vi "test_variance_map.vi"() -> ()   [LabVIEW 2009]
doc: "Copyright (C) 2009, Stepan A. Baranov\nweb: http://www.OCTLab.org/\nemail: stepan@baranov.su"
uses:
  <vilib>/Analysis/NI_AALBase.lvlib
  OCTLib.dll
panel:
  out "vertical radius":i32
  out "error out":errorcluster
  out "horizontal radius":i32
  out "width":i32
  out "height":i32
  in  "Small/Big":bool
  out "loop #":i32
  out "RSM_STAT time":u32
  out "LabView time":u32
  out "RSM_STAT Array":dbl[][](array[numeric])
  out "LabView Array":dbl[][](array[numeric])
  in  "stop":bool
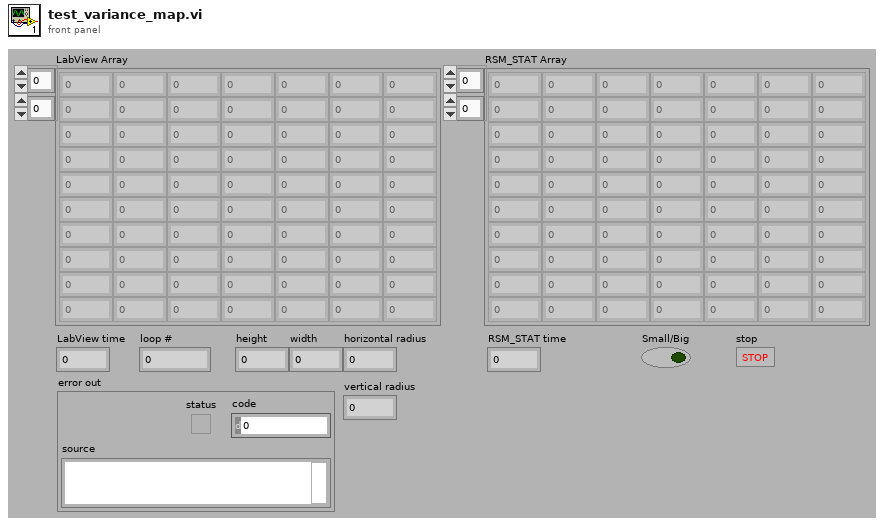
[diagram p1: front panel]
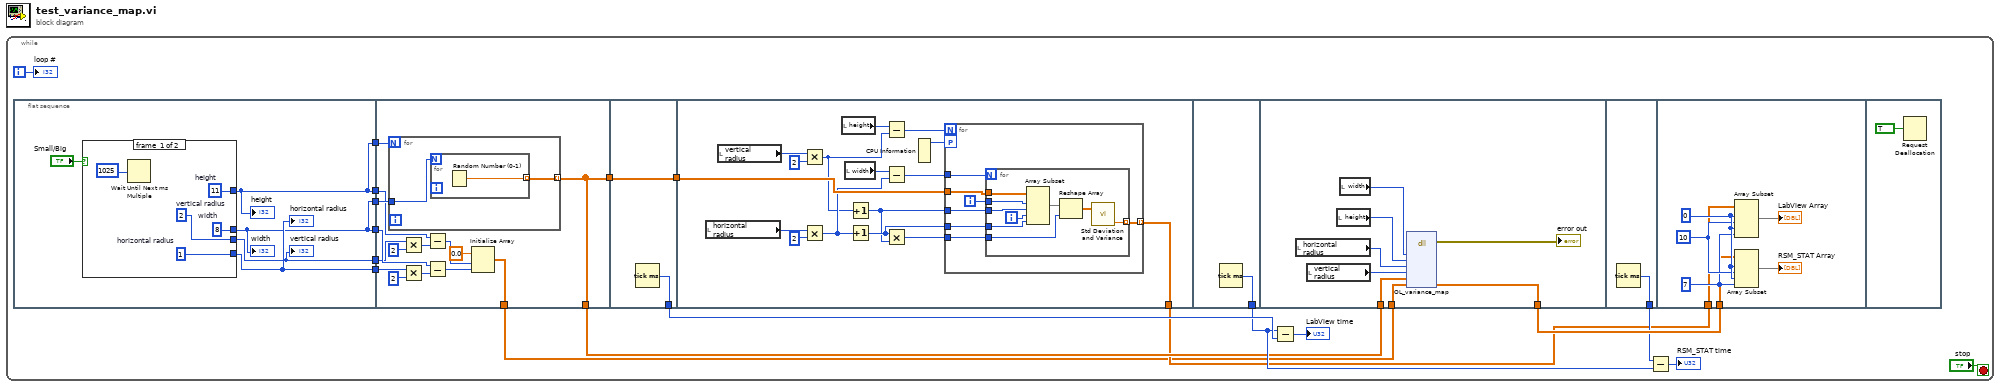
[diagram p0: block diagram]
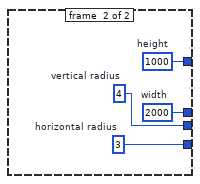
[diagram p2: hidden frame]
diagram:
  n1 = while {
    i -> [w12]
    stop <- "stop" stop-if-true
    n2 = flat-sequence {
      tunnel: [w21] -> w8
      tunnel: [w22] -> w7
      tunnel: [w23] -> w5
      tunnel: [w22] -> w4
      tunnel: [w21] -> w3
      tunnel: [w20] -> w1
      tunnel: [w46] -> w11
      tunnel: [w46] -> w9
      tunnel: w8 -> [w48]
      tunnel: w7 -> [w47]
      tunnel: w5 -> [w44]
      tunnel: w4 -> [w42]
      tunnel: w3 -> [w40]
      tunnel: [w37] -> w2
      tunnel: w1 -> [w35]
      tunnel: [w53] -> w17
      tunnel: [w52] -> w10
      tunnel: w9 -> [w52]
      tunnel: w10 -> [w69]
      tunnel: [w65] -> w6
      tunnel: [w86] -> w14
      tunnel: w11 -> [w93]
      tunnel: [w92] -> w18
      tunnel: w2 -> [w94]
      tunnel: [w95] -> w15
      tunnel: w18 -> [w98]
      tunnel: w6 -> [w97]
      frame #0 {
        n3 = case shown="False" "Small/Big" {
          tunnel: [w27 w33] -> w22
          tunnel: [w28 w32] -> w21
          tunnel: [w29 w31] -> w23
          tunnel: [w25 w30] -> w20
          frame #0 {
            w25 = 2  # vertical radius
            w29 = 1  # horizontal radius
            w28 = 8  # width
            w27 = 11  # height
            n4 = Wait Until Next ms Multiple(millisecond multiple=u32 1025) -> ()  [unwired: 1 out]
          }
          frame #1 {
            w30 = 4  # vertical radius
            w31 = 3  # horizontal radius
            w32 = 2000  # width
            w33 = 1000  # height
          }
        }
        "height" <- w22
        "width" <- w21
        "horizontal radius" <- w23
        "vertical radius" <- w20
      }
      frame #1 {
        n5 = for {
          N: w47 -> [_]
          tunnel: w48 -> [w50]
          tunnel: [w49] -> w46 mode=indexing
          n6 = for {
            N: w50 -> [_]
            tunnel: [w51] -> w49 mode=indexing
            n7 = Random Number (0-1)() -> (number: 0 to 1=w51:dbl)
          }
        }
        n8 = Multiply(x=w35, y=2) -> (x*y=w34:i32)
        n9 = Multiply(x=w44, y=2) -> (x*y=w39:i32)
        n10 = Subtract(x=w42, y=w34) -> (x-y=w41:i32)
        n11 = Subtract(x=w40, y=w39) -> (x-y=w38:i32)
        n12 = Initialize Array(0.0 ("element"), w41, w38) -> (w37:dbl[][])
      }
      frame #2 {
        n13 = Tick Count (ms)() -> (millisecond timer value=w53:u32)
      }
      frame #3 {
        n14 = local read "horizontal radius"() -> (w68:i32)
        n15 = local read "vertical radius"() -> (w57:i32)
        n16 = Multiply(x=w57, y=2) -> (x*y=w55:i32)
        n17 = Multiply(x=w68, y=2) -> (x*y=w61:i32)
        n18 = local read "height"() -> (w64:i32)
        n19 = local read "width"() -> (w62:i32)
        n20 = Increment(x=w55) -> (x+1=w54:i32)
        n21 = Increment(x=w61) -> (x+1=w56:i32)
        n22 = Subtract(x=w64, y=w55) -> (x-y=w63:i32)
        n23 = Subtract(x=w62, y=w61) -> (x-y=w60:i32)
        n24 = Multiply(x=w56, y=w54) -> (x*y=w66:i32)
        n25 = CPU Information() -> (4:w59:i32)  [unwired: 3 out]
        n26 = for {
          N: w63 -> [_]
          tunnel: w69 -> [w75]
          tunnel: w66 -> [w74]
          tunnel: [w73] -> w65 mode=indexing
          tunnel: w56 -> [w72]
          tunnel: w60 -> [w71]
          workers-P: w59 -> [_]
          tunnel: w54 -> [w70]
          i -> [w76]
          n27 = for {
            N: w71 -> [_]
            tunnel: w76 -> [w85]
            tunnel: w75 -> [w83]
            tunnel: w74 -> [w79]
            tunnel: [w77] -> w73 mode=indexing
            tunnel: w72 -> [w82]
            tunnel: w70 -> [w81]
            i -> [w84]
            n28 = Array Subset(array=w83, index (row)=w85, length (row)=w81, index (col)=w84, length (col)=w82) -> (w78:dbl[][])
            n29 = Reshape Array(w78, w79) -> (w80:dbl[])
            n30 = call <vilib>:"Std Deviation and Variance.vi"("X"=w80) -> ("variance"=w77:dbl)  [unwired: 1 in, 2 out]
          }
        }
      }
      frame #4 {
        n31 = Tick Count (ms)() -> (millisecond timer value=w86:u32)
      }
      frame #5 {
        n32 = local read "horizontal radius"() -> (w88:i32)
        n33 = local read "vertical radius"() -> (w87:i32)
        n34 = local read "height"() -> (w90:i32)
        n35 = local read "width"() -> (w91:i32)
        n36 = dll-call lib="OCTLib.dll" fn="OL_variance_map"("width"=w91, "height"=w90, "horizontal radius"=w88, "vertical radius"=w87, "input"=w93, "output"=w94) -> (error out=→"error out":errorcluster, "output"=w92:dbl[][])  [unwired: 9 in, 1 out]
      }
      frame #6 {
        n37 = Tick Count (ms)() -> (millisecond timer value=w95:u32)
      }
      frame #7 {
        w101 = 10 ("length")
        w100 = 7 ("length")
        w102 = 0 ("index")
        n38 = Array Subset(array=w97, index (row)=w102, length (row)=w101, index (col)=w102, length (col)=w100) -> (→"LabView Array":dbl[][])
        n39 = Array Subset(array=w98, index (row)=w102, length (row)=w101, index (col)=w102, length (col)=w100) -> (→"RSM_STAT Array":dbl[][])
      }
      frame #8 {
        n40 = Request Deallocation(TRUE ("flag")) -> ()
      }
    }
    n41 = Subtract(x=w14, y=w17) -> (x-y=→"LabView time":u32)
    n42 = Subtract(x=w15, y=w14) -> (x-y=→"RSM_STAT time":u32)
    "loop #" <- w12
  }
